vi "Number to Proper English text - 0 to 19.vi"(11 "Positive integer <= 19":u16) -> (3 "Integer written in English":string)   [LabVIEW 2021, in "Project Euler.lvlib"]
uses:
  Project Euler.lvlib
panel:
  # "Development\ncontrols/indicators useful for development and testing, but which are not outputs of the VI"
  # "Input\nInputs to the VI"
  # "Output\nOutputs of the VI"
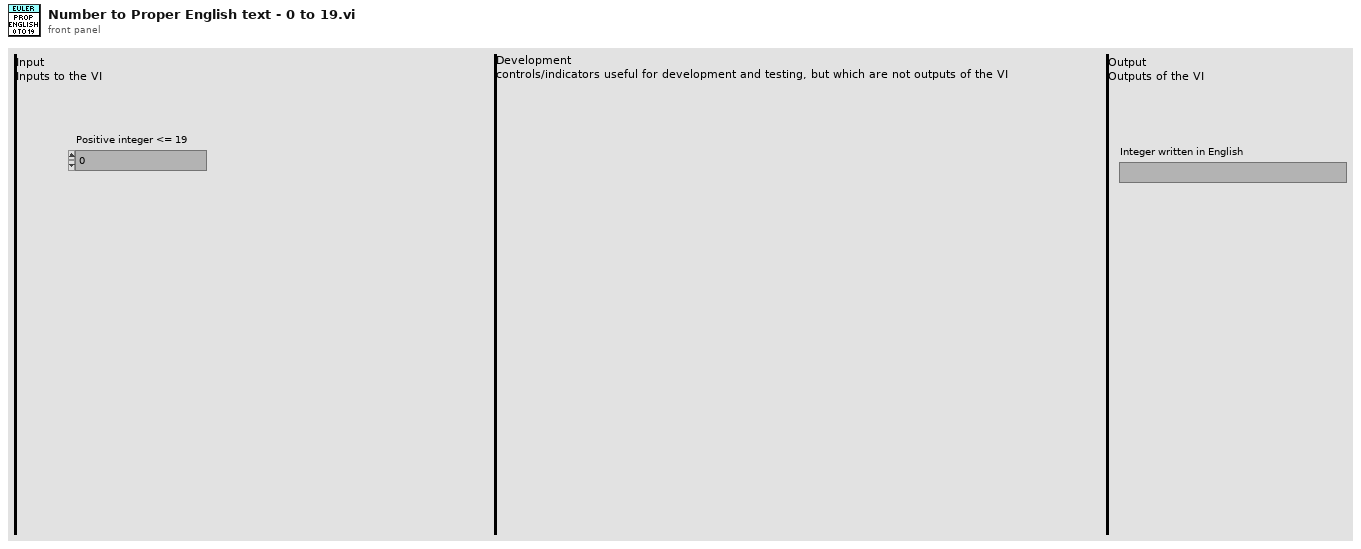
[diagram p1: front panel]
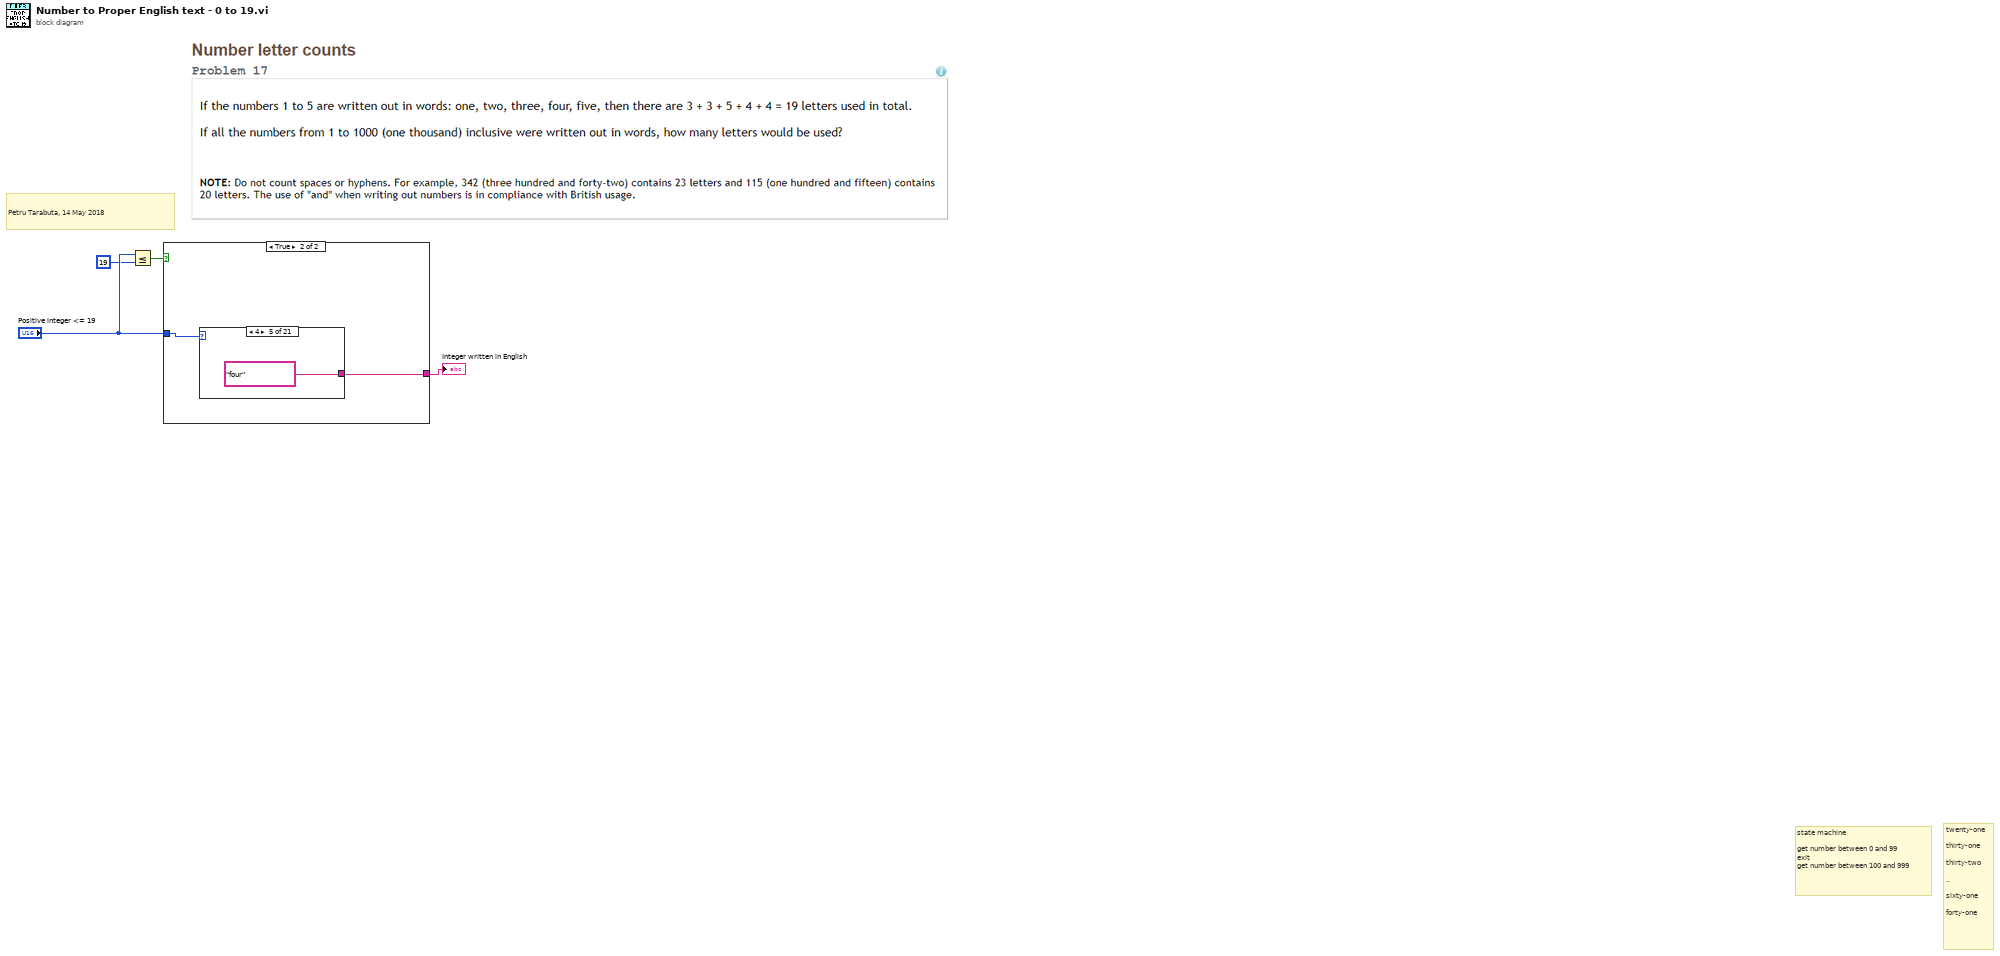
[diagram p0: block diagram]
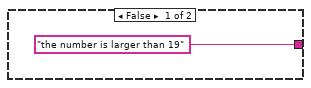
[diagram p2: hidden frame]
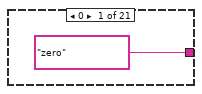
[diagram p3: hidden frame]
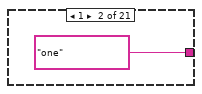
[diagram p4: hidden frame]
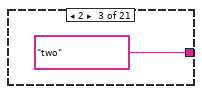
[diagram p5: hidden frame]
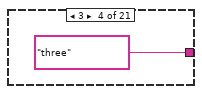
[diagram p6: hidden frame]
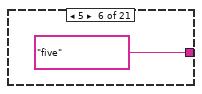
[diagram p7: hidden frame]
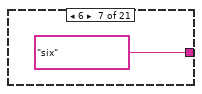
[diagram p8: hidden frame]
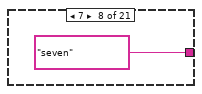
[diagram p9: hidden frame]
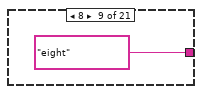
[diagram p10: hidden frame]
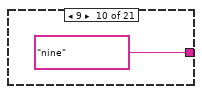
[diagram p11: hidden frame]
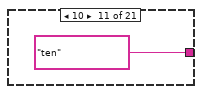
[diagram p12: hidden frame]
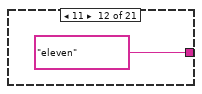
[diagram p13: hidden frame]
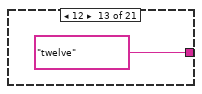
[diagram p14: hidden frame]
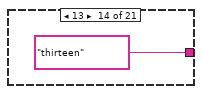
[diagram p15: hidden frame]
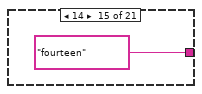
[diagram p16: hidden frame]
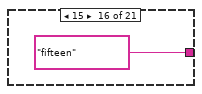
[diagram p17: hidden frame]
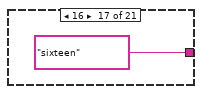
[diagram p18: hidden frame]
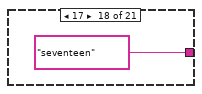
[diagram p19: hidden frame]
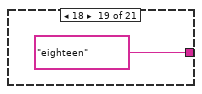
[diagram p20: hidden frame]
diagram:
  # "state machine\n\nget number between 0 and 99\nexit\nget number between 100 and 999"
  # "twenty-one\n\nthirty-one\n\nthirty-two\n\n..\n\nsixty-one\n\nforty-one"
  # "Petru Tarabuta, 14 May 2018"
  n1 = Less Or Equal?(x="Positive integer <= 19", y=u16 19) -> (x <= y?=w1:bool)
  n2 = case shown="True" w1 {
    tunnel: ["the number is larger than 19" w7] -> w4
    tunnel: "Positive integer <= 19" -> [_ w6]
    frame False {
    }
    frame True {
      n3 = case shown="4" w6 {
        tunnel: ["zero" "one" "two" "three" "four" "five" "six" "seven" "eight" "nine" "ten" "eleven" "twelve" "thirteen" "fourteen" "fifteen" "sixteen" "seventeen" "eighteen" "nineteen" "program_flow_error"] -> w7
        frame 0 {
        }
        frame 1 {
        }
        frame 2 {
        }
        frame 3 {
        }
        frame 4 {
        }
        frame 5 {
        }
        frame 6 {
        }
        frame 7 {
        }
        frame 8 {
        }
        frame 9 {
        }
        frame 10 {
        }
        frame 11 {
        }
        frame 12 {
        }
        frame 13 {
        }
        frame 14 {
        }
        frame 15 {
        }
        frame 16 {
        }
        frame 17 {
        }
        frame 18 {
        }
        frame 19 {
        }
        frame Default {
        }
      }
    }
  }
  "Integer written in English" <- w4
